vi "FF_Bkgnd_correction.vi"() -> (0 "Numbers of points":i32[](array[numeric]), 1 "Bkgnd (ppm)":dbl[](array[numeric]))   [LabVIEW 2014]
uses:
  Controls/Analysis_info_cluster.ctl
  Controls/Inst_type.ctl
  Controls/Instrument_Array.ctl
  Controls/Multi_run_mode.ctl
  <vilib>/Analysis/baseanly.llb/Mean (DBL).vi
  Globals/Meas_global.vi
  Globals/Plug_in_data_global.vi
  Globals/Trav_pos_global.vi
  <vilib>/Analysis/NI_AALBase.lvlib
panel:
  out "Number of Samples":i32
  out "Bkgnd c^2 Values":dbl[](array[numeric])
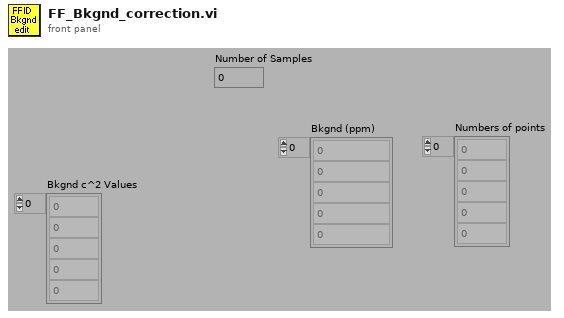
[diagram p1: front panel]
types:
  T1 = cluster{"Weighting":dbl[], "Time (ms)":dbl[], "Voltage":dbl[], "Eng Values":dbl[]}
  T2 = typedef "Analysis_info_cluster.ctl" = cluster{"Colour":u32, "Inst type":T3, "Inst name":string, "Symbol":string, "Code name":string, "Extra Info":string, "Inst Array":T4, "Extra Titles":string[], "Extra Values":string[], "U":dbl, "u^2":dbl, "u^3":dbl, "u^4":dbl, "Skew_u":dbl, "Kurt_u":dbl, "Sd Error in Mean":dbl, "% u'/U":dbl, "X":dbl, "Y":dbl, "Z":dbl, "Timescale integral to 25%":dbl, "Sd Error in Variance":dbl, "Calib File":path, "Calib Constants":dbl[], "Output Position":bool, "Full Stats":bool, "Av Sampling Rate":dbl, "Av No of Samples":dbl, "Total Meas Time (s)":dbl, "ADAM Ch Name":string}
  T3 = typedef "Inst_type.ctl" = enum16{"Propeller anemometer", "Raw voltage", "Pressure Transducer", "Pitot-static tube", "Preston tube", "Hot wire", "Cross wire 1", "Cross wire 2", "Generic Linear", "Generic Polynomial", "Generic BackPoly", "Fast FID", "Thermocouple", "Cold wire", "Pulsed Wire", "LDA Vel", "LDA Tran time", "LDA Arr time", "Microphone"}
  T4 = typedef "Instrument_Array.ctl" = enum16{"PWA", "LDA", "Analogue"}
  T5 = typedef "Multi_run_mode.ctl" = enum16{"Move Traverse Only", "Set Tunnel Speed Only", "Set Source Only", "Set Measurement Conditions", "Single Measurement", "Vertical Profile", "Lateral Profile", "Longitudinal Profile", "Explore Volume", "Multi-Axis Profile", "Auto Calibrate", "Meas Fast FID Bkgnd", "Check Beam Power", "Scanning Valve Measurement", "Run VI Named:", "Set ADAM Ch", "Wait (minutes)", "Send Message", "Synchronize With:", "Fall Back to this Row", "Turn Off Row Repeating", "Blank Row", "Traverse 3D Volume"}
  T6 = typedef "Time_Trace_Cluster.ctl" = cluster{"Weighting":dbl[], "Time (s)":dbl[], "Voltage":dbl[], "Eng Values":dbl[]}
  T7 = cluster{"Weighting":dbl[], "Time (ms)":dbl[], "Voltage":dbl[], "Eng Values":dbl[]}[]
  T8 = typedef "Post_Process.ctl" = enum16{"Take New Data", "Post Process Raw Data File"}
  T9 = typedef "Traverse_cluster.ctl" = cluster{"Start X":sgl, "Start Y":sgl, "Start Z":sgl, "End X":sgl, "End Y":sgl, "End Z":sgl, "No. of pts.":i32, "Spacing":T10, "Filename":path, "Tunnel Speed":dbl, "Averaging time (min)":dbl, "Extra Commands":string, "Specific Arguments":string, "Emission Rate (l/min)":dbl, "Trace Gas Concentration (%)":dbl, "Density Ratio":string, "Comments":string, "Row No":i32, "Row Type Selector":T5, "Completion time":string, "Row Duration (mins)":dbl, "No. of Valid pts.":i32, "Meas Setup File":string}
  T10 = typedef "Spacing.ctl" = enum16{"Linear", "Log", "Gauss", "Specified", "N/A"}
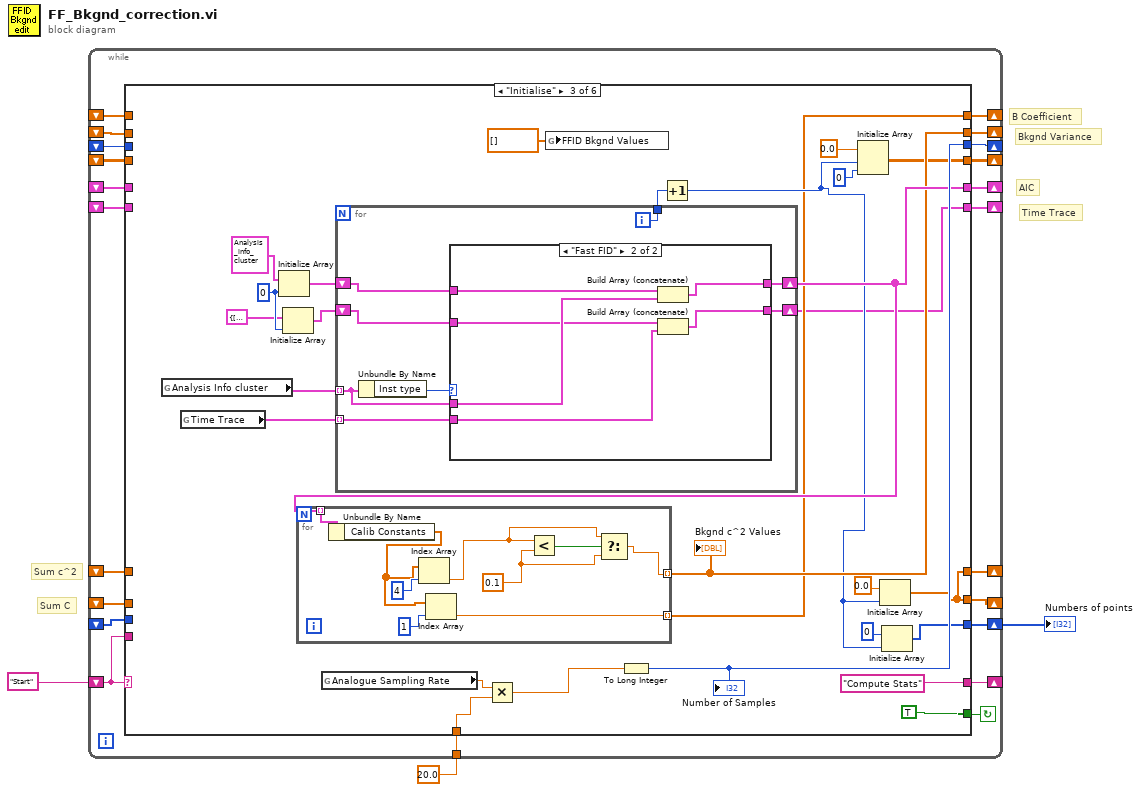
[diagram p0: block diagram]
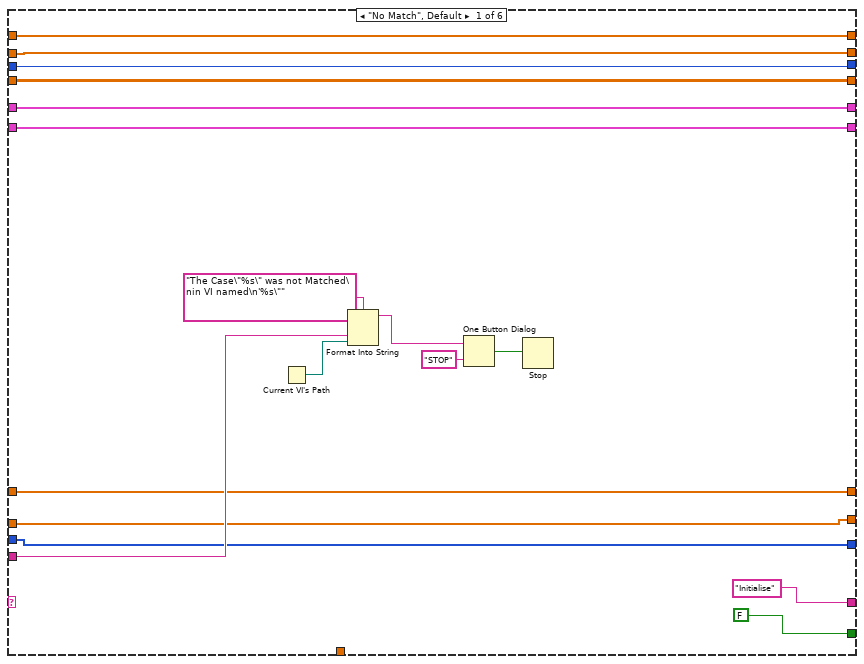
[diagram p2: hidden frame]
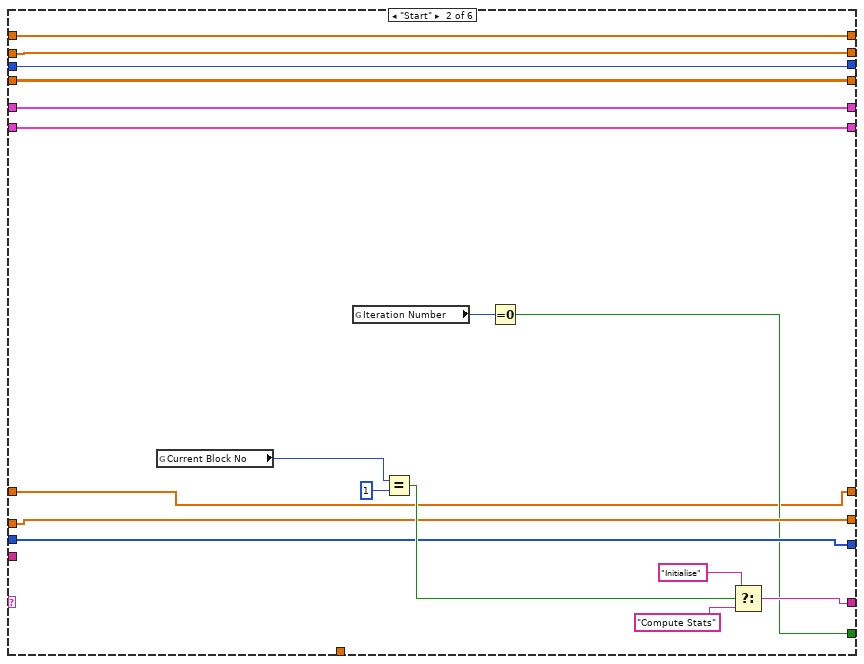
[diagram p3: hidden frame]
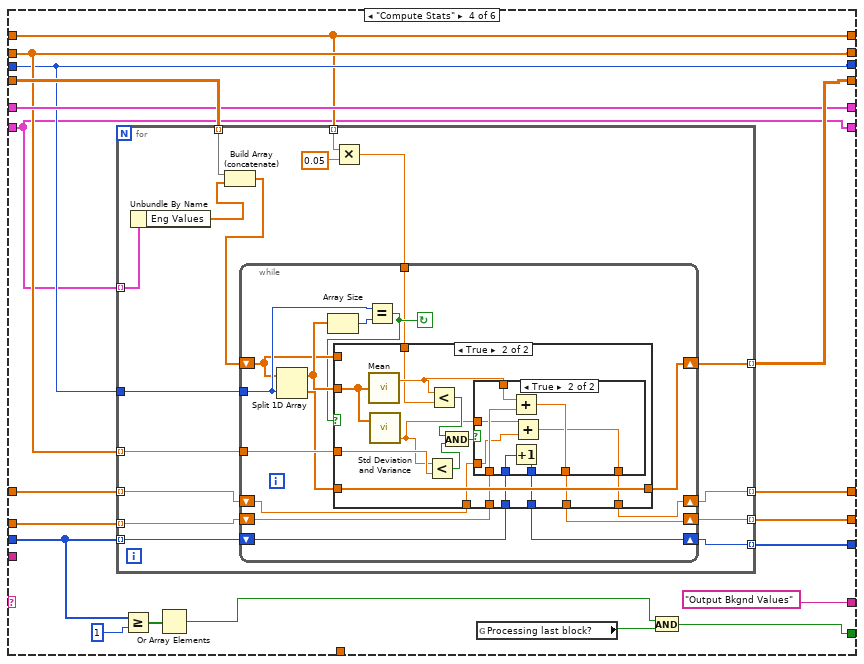
[diagram p5: hidden frame]
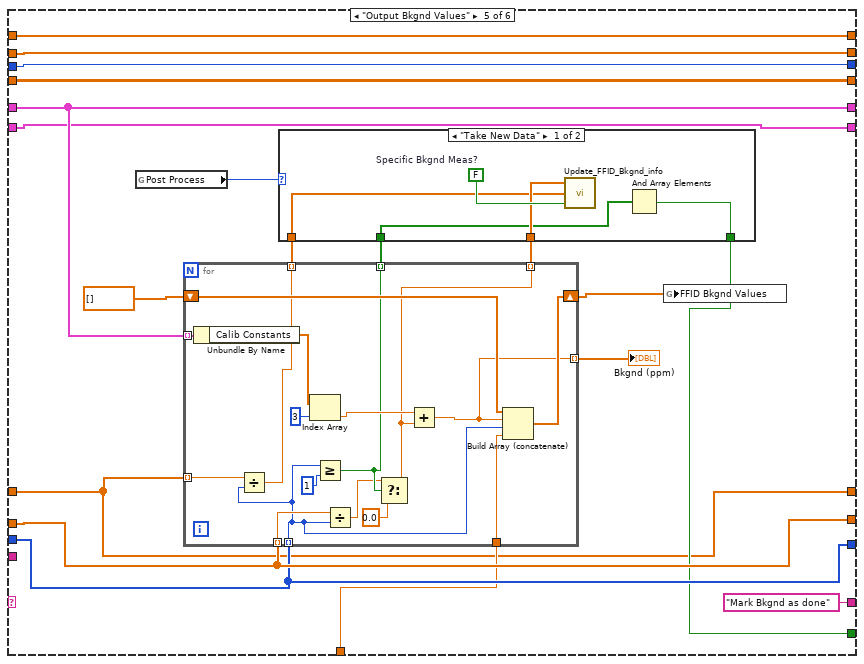
[diagram p8: hidden frame]
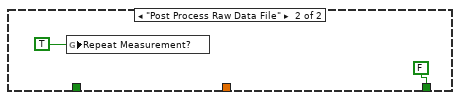
[diagram p9: hidden frame]
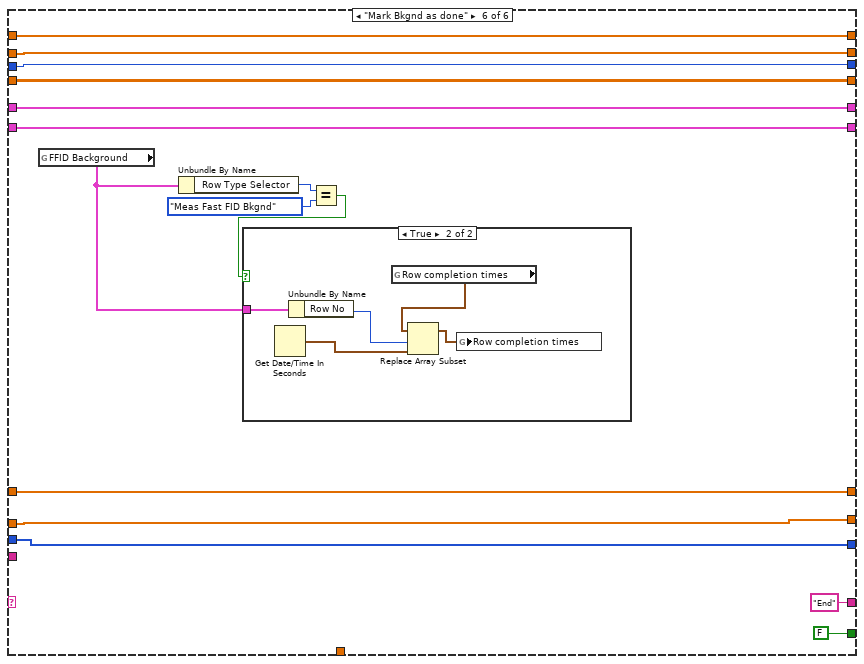
[diagram p10: hidden frame]
diagram:
  # "Time Trace"
  # "AIC"
  # "Bkgnd Variance"
  # "B Coefficient"
  # "Sum C"
  # "Sum c^2"
  n1 = while {
    shift-left: "Start" -> [w23]
    shift-right: [w24] -> _
    shift-right: [w22] -> _
    shift-left: _ -> [w20]
    shift-right: [w18] -> _
    shift-left: _ -> [w19]
    shift-right: [w21] -> _
    shift-left: _ -> [w17]
    shift-right: [w16] -> _
    shift-left: _ -> [w15]
    shift-right: [w13] -> _
    shift-left: _ -> [w14]
    shift-right: [w12] -> w2
    shift-left: _ -> [w11]
    tunnel: 20.0 ("y") -> [w10]
    shift-right: [w9] -> _
    shift-left: _ -> [w8]
    shift-right: [w6] -> _
    shift-left: _ -> [w7]
    shift-right: [w5] -> _
    shift-left: _ -> [w4]
    stop <- w25 continue-if-true
    n2 = case shown="\"Initialise\"" w23 {
      tunnel: [FALSE w46 TRUE w121 w199 FALSE] -> w25
      tunnel: ["Initialise" w56 "Compute Stats" "Output Bkgnd Values" "Mark Bkgnd as done" ("f") "End" ("f")] -> w24
      tunnel: w23 -> [w37 _ _ _ _ _]
      tunnel: [w31 w51 w80 w128 w205 w244] -> w22
      tunnel: [w33 w53 w81 w126 w207 w246] -> w21
      tunnel: w20 -> [w31 w51 _ w128 w205 w244]
      tunnel: w19 -> [w32 w52 _ w130 w206 w245]
      tunnel: [w32 w52 w75 w129 w206 w245] -> w18
      tunnel: w17 -> [w33 w53 _ w126 w207 w246]
      tunnel: [w34 w54 w79 w127 w208 w247] -> w16
      tunnel: w15 -> [w34 w54 _ w127 w208 w247]
      tunnel: w14 -> [w30 w50 _ w125 w210 w249]
      tunnel: [w30 w50 w67 w124 w210 w249] -> w13
      tunnel: [w29 w49 w72 w123 w209 w248] -> w12
      tunnel: w11 -> [w29 w49 _ w119 w209 w248]
      tunnel: w10 -> [_ _ w69 _ w203 _]
      tunnel: [w28 w45 w68 w115 w195 w237] -> w9
      tunnel: w8 -> [w28 w45 _ w115 w195 w237]
      tunnel: w7 -> [w27 w44 _ w114 w194 w236]
      tunnel: [w27 w44 w67 w113 w194 w236] -> w6
      tunnel: [w26 w43 w60 w112 w192 w235] -> w5
      tunnel: w4 -> [w26 w43 _ w112 w192 w235]
      frame "No Match", Default {
        n3 = Current VI's Path() -> (path=w36:path)
        n4 = Format Into String(format string="The Case\"%s\" was not Matched\nin VI named\n'%s\"" ("Format String"), w37, w36) -> (resulting string=w40:string)  [unwired: 2 in, 1 out]
        n5 = One Button Dialog(message=w40, button name ("OK")="STOP") -> (true=w38:bool)
        n6 = Stop(stop? (T)=w38) -> ()
      }
      frame "Start" {
        n7 = global read "Meas_global.vi" "Current Block No"() -> (w48:i32)
        n8 = global read "Meas_global.vi" "Iteration Number"() -> (w47:i32)
        n9 = Equal?(x=w48, y=1) -> (x = y?=w57:bool)
        n10 = Equal To 0?(x=w47) -> (x = 0?=w46:bool)
        n11 = Select(t="Initialise", s=w57, f="Compute Stats") -> (s? t:f=w56:string)
      }
      frame "Initialise" {
        w62 = 0 ("dimension size")
        n12 = global read "Meas_global.vi" "Analysis Info cluster"() -> (w84:T2[])
        n13 = global read "Meas_global.vi" "Time Trace"() -> (w64:T6[])
        n14 = Initialize Array(T2 {"Colour"=0, "Inst type"=enum."Pitot-static tube", "Inst name"="Manometer voltage", "Symbol"="U", "Code name"="", "Extra Info"="U", "Inst Array"=enum."PWA", "Extra Titles"=[], "Extra Values"=[], "U"=0.0, "u^2"=0.0, "u^3"=0.0, "u^4"=0.0, "Skew_u"=0.0, "Kurt_u"=0.0, "Sd Error in Mean"=0.0, "% u'/U"=0.0, "X"=0.0, "Y"=0.0, "Z"=0.0, "Timescale integral to 25%"=0.0, "Sd Error in Variance"=0.0, "Calib File"=path "", "Calib Constants"=[], "Output Position"=FALSE, "Full Stats"=FALSE, "Av Sampling Rate"=0.0, "Av No of Samples"=0.0, "Total Meas Time (s)"=0.0, "ADAM Ch Name"=""} ("Analysis_info_cluster"), w62) -> (w65:T2[])
        n15 = Initialize Array(T1 {"Weighting"=[], "Time (ms)"=[], "Voltage"=[], "Eng Values"=[]} ("Time Trace"), w62) -> (w63:T7)
        n16 = global read "Meas_global.vi" "Analogue Sampling Rate"() -> (w83:dbl)
        n17 = for {
          tunnel: w84 -> [w99] mode=indexing
          shift-right: [w101] -> w80
          shift-left: w65 -> [w102]
          tunnel: [w100] -> w77
          tunnel: w64 -> [w98] mode=indexing
          shift-right: [w96] -> w60
          shift-left: w63 -> [w97]
          i -> [w100]
          n18 = Unbundle By Name(w99) -> ("Inst type"=w103:T3)
          n19 = case shown="\"Fast FID\"" w103 {
            tunnel: w102 -> [w105 w111]
            tunnel: w99 -> [_ w110]
            tunnel: [w105 w109] -> w101
            tunnel: w98 -> [_ w108]
            tunnel: w97 -> [w104 w107]
            tunnel: [w104 w106] -> w96
            frame "Propeller anemometer", Default {
            }
            frame "Fast FID" {
              n20 = Build Array (concatenate)(w111, w110) -> (w109:T2[])
              n21 = Build Array (concatenate)(w107, w108) -> (w106:T6[])
            }
          }
        }
        n22 = for {
          tunnel: w80 -> [w88] mode=indexing
          tunnel: [w89] -> w79 mode=indexing
          tunnel: [w93] -> w68 mode=indexing
          w90 = 0.1 ("y")
          n23 = Unbundle By Name(w88) -> ("Calib Constants"=w87:dbl[])
          n24 = Index Array(array=w87, index=4) -> (element=w91:dbl)
          n25 = Index Array(array=w87, index=1) -> (element=w93:dbl)
          n26 = Less?(x=w91, y=w90) -> (x < y?=w92:bool)
          n27 = Select(t=w91, s=w92, f=w90) -> (s? t:f=w89:dbl)
        }
        "Bkgnd c^2 Values" <- w79
        n28 = Multiply(x=w83, y=w69) -> (x*y=w82:dbl)
        n29 = global write "Plug_in_data_global.vi" "FFID Bkgnd Values"(dbl[] [] ("FFID Bkgnd Values")) -> ()
        n30 = To Long Integer(number=w82) -> (32bit integer=w81:i32)
        "Number of Samples" <- w81
        n31 = Increment(x=w77) -> (x+1=w71:i32)
        n32 = Initialize Array(0.0, w71, 0 ("dimension size")) -> (w75:dbl[][])
        n33 = Initialize Array(0.0, w71) -> (w67:dbl[])
        n34 = Initialize Array(0, w71) -> (w72:i32[])
      }
      frame "Compute Stats" {
        n35 = for {
          tunnel: w130 -> [w146] mode=indexing
          tunnel: w126 -> [w144]
          tunnel: w127 -> [w143] mode=indexing
          tunnel: [w142] -> w129 mode=indexing
          tunnel: w125 -> [w141] mode=indexing
          tunnel: [w140] -> w124 mode=indexing
          tunnel: w119 -> [w139] mode=indexing
          tunnel: [w138] -> w123 mode=indexing
          tunnel: w115 -> [w136] mode=indexing
          tunnel: w114 -> [w134] mode=indexing
          tunnel: [w133] -> w113 mode=indexing
          tunnel: w112 -> [w131] mode=indexing
          n36 = Unbundle By Name(w131) -> ("Eng Values"=w132:dbl[])
          n37 = Build Array (concatenate)(w146, w132) -> (w145:dbl[])
          n38 = Multiply(x=w136, y=0.05) -> (x*y=w135:dbl)
          n39 = while {
            shift-right: [w157] -> w142
            shift-left: w145 -> [w156]
            tunnel: w144 -> [w158]
            tunnel: w143 -> [w161]
            shift-right: [w152] -> w140
            shift-left: w141 -> [w153]
            shift-right: [w151] -> w138
            shift-left: w139 -> [w150]
            tunnel: w135 -> [w149]
            shift-right: [w148] -> w133
            shift-left: w134 -> [w147]
            stop <- w154 continue-if-true
            n40 = Split 1D Array(array=w156, index=w158) -> (first subarray=w160:dbl[], second subarray=w155:dbl[])
            n41 = Array Size(array=w160) -> (size(s)=w159:i32)
            n42 = Equal?(x=w158, y=w159) -> (x = y?=w154:bool)
            n43 = case shown="True" w154 {
              tunnel: w161 -> [_ w180]
              tunnel: w160 -> [_ w179]
              tunnel: [w165 w178] -> w157
              tunnel: w156 -> [w165 _]
              tunnel: w155 -> [_ w178]
              tunnel: w153 -> [w164 w177]
              tunnel: [w164 w176] -> w152
              tunnel: [w163 w171] -> w151
              tunnel: w150 -> [w163 w170]
              tunnel: w149 -> [_ w169]
              tunnel: [w162 w168] -> w148
              tunnel: w147 -> [w162 w166]
              frame False {
              }
              frame True {
                n44 = call-poly <vilib>:"Mean.vi"("X"=w179) -> ("mean"=w175:dbl)  [unwired: 1 out]
                n45 = call <vilib>:"Std Deviation and Variance.vi"("X"=w179) -> ("variance"=w167:dbl)  [unwired: 1 in, 2 out]
                n46 = Less?(x=w167, y=w180) -> (x < y?=w173:bool)
                n47 = Less?(x=w175, y=w169) -> (x < y?=w172:bool)
                n48 = And(x=w172, y=w173) -> (x .and. y?=w174:bool)
                n49 = case shown="True" w174 {
                  tunnel: w177 -> [w183 w191]
                  tunnel: [w183 w190] -> w176
                  tunnel: w175 -> [_ w187]
                  tunnel: [w182 w189] -> w171
                  tunnel: w170 -> [w182 w188]
                  tunnel: [w181 w186] -> w168
                  tunnel: w167 -> [_ w185]
                  tunnel: w166 -> [w181 w184]
                  frame False {
                  }
                  frame True {
                    n50 = Add(x=w187, y=w191) -> (x+y=w190:dbl)
                    n51 = Increment(x=w188) -> (x+1=w189:i32)
                    n52 = Add(x=w185, y=w184) -> (x+y=w186:dbl)
                  }
                }
              }
            }
          }
        }
        n53 = Greater Or Equal?(x=w119, y=1) -> (x >= y?=w118:bool[])
        n54 = Or Array Elements(Boolean array=w118) -> (logical OR=w117:bool)
        n55 = global read "Meas_global.vi" "Processing last block?"() -> (w122:bool)
        n56 = And(x=w117, y=w122) -> (x .and. y?=w121:bool)
      }
      frame "Output Bkgnd Values" {
        n57 = global read "Meas_global.vi" "Post Process"() -> (w201:T8)
        n58 = for {
          tunnel: w205 -> [w219] mode=indexing
          tunnel: w210 -> [w232] mode=indexing
          tunnel: w209 -> [w222] mode=indexing
          tunnel: w203 -> [w230]
          shift-right: [w229] -> w200
          shift-left: dbl[] [] -> [w228]
          tunnel: [w226] -> w198 mode=indexing
          tunnel: [w227] -> w197 mode=indexing
          tunnel: [w223] -> w196 mode=indexing
          tunnel: w194 -> [w221] mode=indexing
          tunnel: [w220] -> w193 mode=indexing
          n59 = Unbundle By Name(w219) -> ("Calib Constants"=w218:dbl[])
          n60 = Divide(x=w221, y=w222) -> (x/y=w220:dbl)
          n61 = Index Array(array=w218, index=3 ("Index")) -> (element=w233:dbl)
          n62 = Greater Or Equal?(x=w222, y=1) -> (x >= y?=w226:bool)
          n63 = Divide(x=w232, y=w222) -> (x/y=w225:dbl)
          n64 = Select(t=w225, s=w226, f=0.0) -> (s? t:f=w223:dbl)
          n65 = Add(x=w233, y=w223) -> (x+y=w227:dbl)
          n66 = Build Array (concatenate)(w228, w227, w222, w230) -> (w229:dbl[])
        }
        "Bkgnd (ppm)" <- w197
        n67 = case shown="\"Take New Data\"" w201 {
          tunnel: w196 -> [w214 _]
          tunnel: [w212 FALSE] -> w199
          tunnel: w198 -> [w213 _]
          tunnel: w193 -> [w211 _]
          frame "Take New Data" {
            w215 = FALSE  # Specific Bkgnd Meas?
            n68 = call "Update_FFID_Bkgnd_info.vi"("Specific Bkgnd Meas?"=w215, "c^2 (ppm^2)"=w211, "C (ppm)"=w214) -> ()  [unwired: 1 in]
            n69 = And Array Elements(Boolean array=w213) -> (logical AND=w212:bool)
          }
          frame "Post Process Raw Data File" {
            n70 = global write "Meas_global.vi" "Repeat Measurement?"(TRUE ("Repeat Measurement?")) -> ()
          }
        }
        n71 = global write "Plug_in_data_global.vi" "FFID Bkgnd Values"(w200) -> ()
      }
      frame "Mark Bkgnd as done" {
        n72 = global read "Trav_pos_global.vi" "FFID Background"() -> (w239:T9)
        n73 = Unbundle By Name(w239) -> ("Row Type Selector"=w241:T5)
        n74 = Equal?(x=w241, y=Multi_run_mode."Meas Fast FID Bkgnd" ("Row Type Selector")) -> (x = y?=w238:bool)
        n75 = case shown="True" w238 {
          tunnel: w239 -> [_ w254]
          frame False {
          }
          frame True {
            n76 = Get Date/Time In Seconds() -> (seconds since 1Jan1904=w250:timestamp)
            n77 = Unbundle By Name(w254) -> ("Row No"=w253:i32)
            n78 = global read "Trav_pos_global.vi" "Row completion times"() -> (w252:timestamp[])
            n79 = Replace Array Subset(array=w252, new element=w250, index=w253) -> (w251:timestamp[])
            n80 = global write "Trav_pos_global.vi" "Row completion times"(w251) -> ()
          }
        }
      }
    }
  }
  "Numbers of points" <- w2
